vi "Write State to Config.vi"(8 "error in (no error)":errorcluster, 10 "Command":T1, 11 "Plugin Name":string) -> (0 "error out":errorcluster)   [LabVIEW 2021, in "CIFLogs.lvlib"]
uses:
  CIFLogs.lvlib
  Typedef/Plugin State Commands.ctl
  Typedef/Message Type.ctl
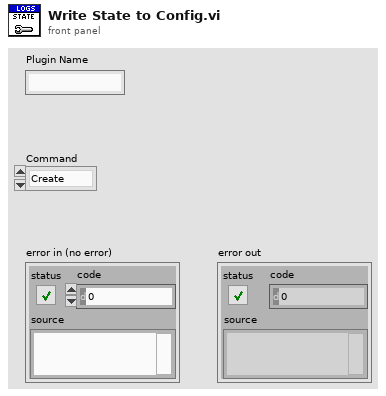
[diagram p1: front panel]
types:
  T1 = typedef "Plugin State Commands.ctl" = enum16{"Create", "Configure", "Run", "Pause", "Destroy"}
  T2 = typedef "CIFLogs.lvlib/Message Type.ctl" = enum16{"Error", "Information", "Print Terminal", "Configuration"}
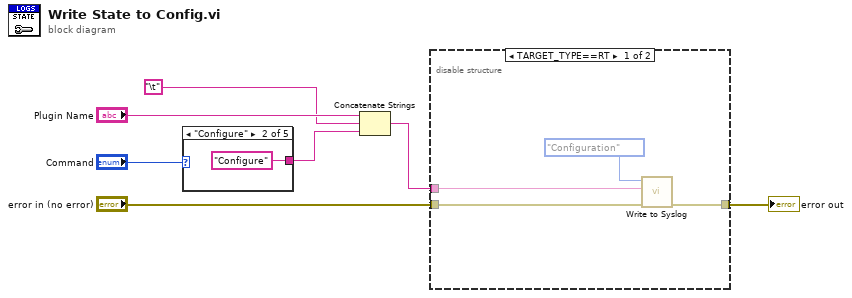
[diagram p0: block diagram]
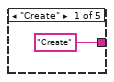
[diagram p2: hidden frame]
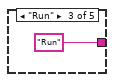
[diagram p3: hidden frame]
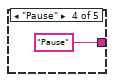
[diagram p4: hidden frame]
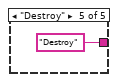
[diagram p5: hidden frame]
diagram:
  n1 = case shown="\"Configure\"" "Command" {
    tunnel: ["Create" "Configure" "Run" "Pause" "Destroy"] -> w1
    frame "Create" {
    }
    frame "Configure" {
    }
    frame "Run" {
    }
    frame "Pause" {
    }
    frame "Destroy" {
    }
  }
  n2 = Concatenate Strings("Plugin Name", "\t", w1) -> (w3:string)
  n3 = disable-structure shown="TARGET_TYPE==RT" {
    disable-tunnel: "error in (no error)" -> [w16 _]
    disable-tunnel: [w15 _] -> w6
    disable-tunnel: w3 -> [w13 _]
    frame condition #0 {
      n4 = call "Write to Syslog.vi"("error in (no error)"=w16, "message"=w13, "CIF Message Type"=Message_Type."Configuration") -> ("error out"=w15:errorcluster)  [unwired: 8 in]
    }
    frame condition #1 (active) {
    }
  }
  "error out" <- w6
